vi "LiftV2.vi"() -> ()   [LabVIEW 2025]
panel:
  in  "Floor 4 CALL":bool caption="Floor 1"
  in  "Floor 3 CALL":bool caption="Floor 1"
  in  "Floor 2 CALL":bool caption="Floor 1"
  in  "Floor 1 CALL":bool caption="Floor 1"
  in  "STOP 2":bool caption="Floor 1"
  in  "STOP":bool caption="Floor 1"
  in  "Floor 4":bool
  in  "Floor 3":bool
  in  "Floor 2":bool
  out "2 LED":bool
  out "Floor":i32
  in  "Floor 1":bool
  out "On/Off":bool
  out "s? t:f 4":i32
  out "s? t:f 3":i32
  out "s? t:f 2":i32
  out "s? t:f":i32
  out "UD2":bool
  out "target_pos":i32
  out "Current_Pos":i32
  out "Lift":bool
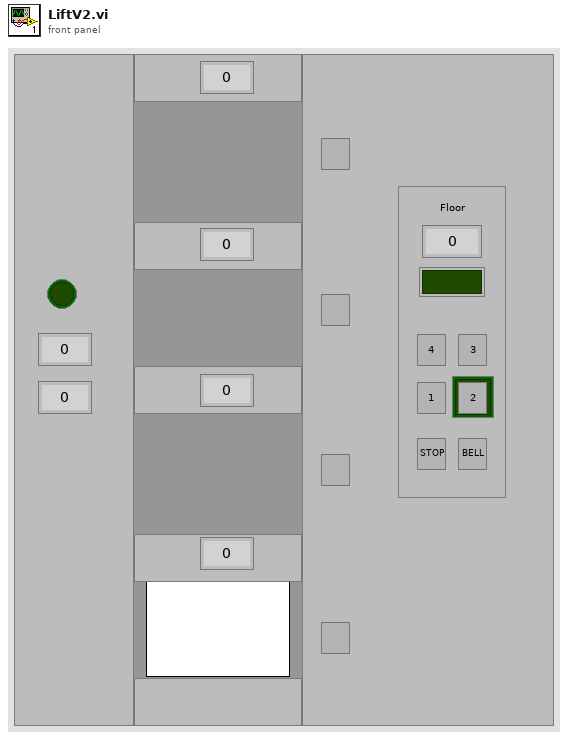
[diagram p1: front panel]
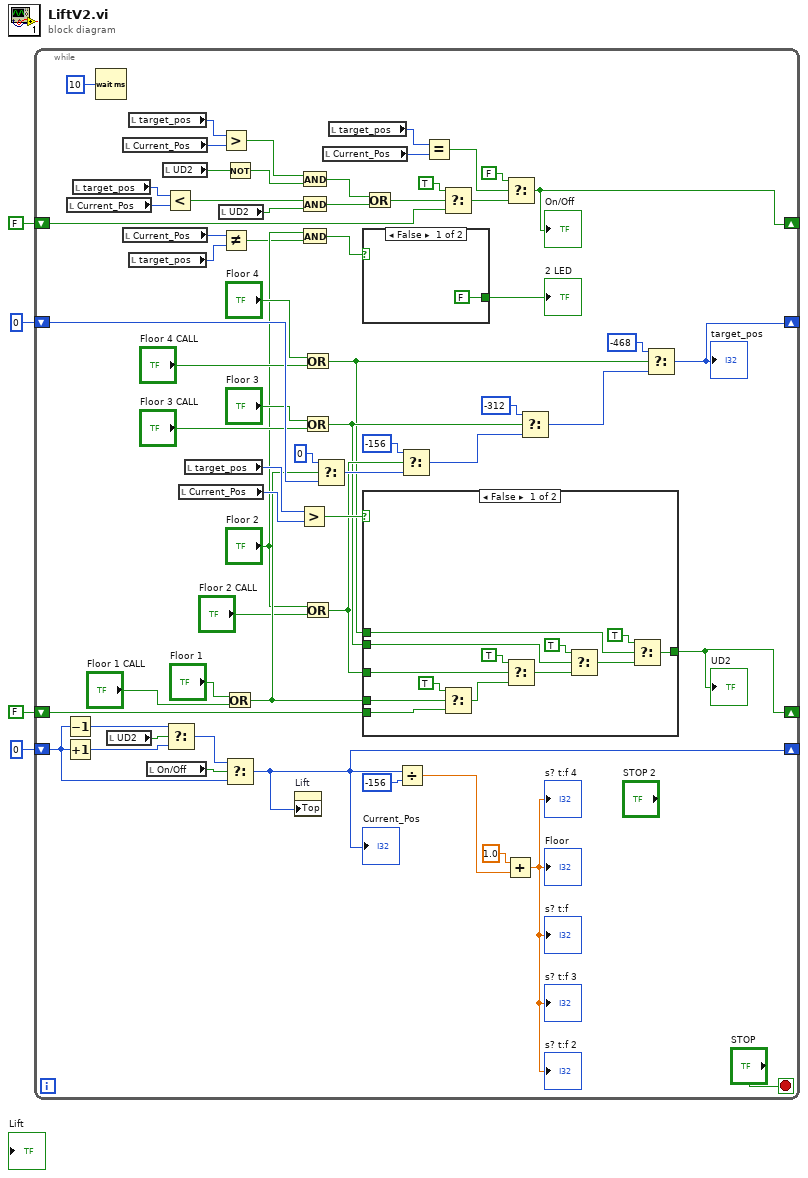
[diagram p0: block diagram]
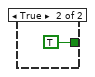
[diagram p2: hidden frame]
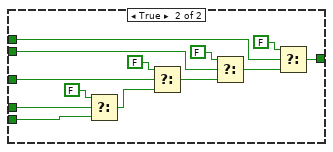
[diagram p3: hidden frame]
diagram:
  n1 = while {
    shift-right: [w27] -> _
    shift-left: 0 -> [w65]
    shift-right: [w57] -> _
    shift-left: FALSE -> [w62]
    shift-right: [w34] -> _
    shift-left: 0 -> [w36]
    shift-right: [w32] -> _
    shift-left: FALSE -> [w33]
    stop <- "STOP" stop-if-true
    n2 = Decrement(x=w65) -> (x-1=w68:i32)
    n3 = Increment(x=w65) -> (x+1=w67:i32)
    n4 = local read "Current_Pos"() -> (w58:i32)
    n5 = local read "target_pos"() -> (w30:i32)
    n6 = Wait (ms)(milliseconds to wait=u32 10) -> ()  [unwired: 1 out]
    n7 = local read "UD2"() -> (w31:bool)
    n8 = local read "Current_Pos"() -> (w51:i32)
    n9 = local read "Current_Pos"() -> (w9:i32)
    n10 = local read "target_pos"() -> (w52:i32)
    n11 = local read "target_pos"() -> (w10:i32)
    n12 = local read "On/Off"() -> (w64:bool)
    n13 = local read "UD2"() -> (w49:bool)
    n14 = Less?(x=w30, y=w58) -> (x < y?=w56:bool)
    n15 = Select(t=w68, s=w31, f=w67) -> (s? t:f=w66:i32)
    n16 = local read "Current_Pos"() -> (w45:i32)
    n17 = local read "target_pos"() -> (w44:i32)
    n18 = local read "UD2"() -> (w28:bool)
    n19 = Greater?(x=w52, y=w51) -> (0:w50:bool)
    n20 = Not Equal?(x=w9, y=w10) -> (x != y?=w7:bool)
    n21 = Not(x=w49) -> (.not. x?=w48:bool)
    n22 = Or(x="Floor 1", y="Floor 1 CALL") -> (x .or. y?=w19:bool)
    n23 = Select(t=w66, s=w64, f=w65) -> (s? t:f=w27:i32)
    "Current_Pos" <- w27
    n24 = property on="Lift" class="Bool (strict)"("Top"=w27) -> ()  [unwired: 2 in, 2 out]
    n25 = Greater?(x=w44, y=w45) -> (0:w43:bool)
    n26 = And(x=w50, y=w48) -> (x .and. y?=w46:bool)
    n27 = And(x=w56, y=w28) -> (x .and. y?=w55:bool)
    n28 = And(x="Floor 2", y=w7) -> (x .and. y?=w6:bool)
    n29 = Or(x="Floor 4", y="Floor 4 CALL") -> (x .or. y?=w11:bool)
    n30 = Or(x="Floor 3", y="Floor 3 CALL") -> (x .or. y?=w14:bool)
    n31 = Or(x="Floor 2", y="Floor 2 CALL") -> (x .or. y?=w17:bool)
    n32 = Select(t=0, s=w19, f=w36) -> (s? t:f=w40:i32)
    n33 = local read "Current_Pos"() -> (w54:i32)
    n34 = local read "target_pos"() -> (w29:i32)
    n35 = case shown="False" w6 {
      tunnel: [FALSE ("2 LED") TRUE ("2 LED")] -> w5
      frame False {
      }
      frame True {
      }
    }
    "2 LED" <- w5
    n36 = case shown="False" w43 {
      tunnel: w33 -> [w76 w96]
      tunnel: w19 -> [w75 w88]
      tunnel: w17 -> [w71 w84]
      tunnel: w14 -> [w72 w87]
      tunnel: w11 -> [w74 w86]
      tunnel: [w73 w85] -> w32
      frame False {
        n37 = Select(t=TRUE, s=w75, f=w76) -> (s? t:f=w83:bool)
        n38 = Select(t=TRUE, s=w71, f=w83) -> (s? t:f=w82:bool)
        n39 = Select(t=TRUE, s=w72, f=w82) -> (s? t:f=w81:bool)
        n40 = Select(t=TRUE, s=w74, f=w81) -> (s? t:f=w73:bool)
      }
      frame True {
        n41 = Select(t=FALSE, s=w88, f=w96) -> (s? t:f=w95:bool)
        n42 = Select(t=FALSE, s=w84, f=w95) -> (s? t:f=w94:bool)
        n43 = Select(t=FALSE, s=w87, f=w94) -> (s? t:f=w93:bool)
        n44 = Select(t=FALSE, s=w86, f=w93) -> (s? t:f=w85:bool)
      }
    }
    "UD2" <- w32
    n45 = Or(x=w46, y=w55) -> (x .or. y?=w47:bool)
    n46 = Divide(x=w27, y=-156 ("x")) -> (x/y=w25:dbl)
    n47 = Select(t=-156, s=w17, f=w40) -> (s? t:f=w41:i32)
    n48 = Equal?(x=w29, y=w54) -> (x = y?=w53:bool)
    n49 = Select(t=TRUE, s=w47, f=w62) -> (s? t:f=w61:bool)
    n50 = Add(x=1.0, y=w25) -> (x+y=→"s? t:f" →"s? t:f 2" →"s? t:f 3" →"s? t:f 4" →"Floor":dbl)
    n51 = Select(t=FALSE, s=w53, f=w61) -> (s? t:f=w57:bool)
    "On/Off" <- w57
    n52 = Select(t=-312, s=w14, f=w41) -> (s? t:f=w42:i32)
    n53 = Select(t=-468, s=w11, f=w42) -> (s? t:f=w34:i32)
    "target_pos" <- w34
  }
